vi "PID_Tank.vi"() -> ()   [LabVIEW 2014]
uses:
  <vilib>/Simulation/Scripting/Companion Diagram/SimConfigNode/SimParams.ctl
  <vilib>/Simulation/Scripting/Companion Diagram/SimConfigNode/_simSolvers.ctl
  <vilib>/Simulation/Implementation/Shared/SIMSCR Execution Mode.ctl
  <vilib>/Simulation/Param Hierarchy/Typedefs/SIMPH Param Control Actions.ctl
  <vilib>/Simulation/Implementation/Shared/SIM limit type.ctl
  <vilib>/Simulation/Implementation/Shared/NILVSim_ParamChanged.vi
  <vilib>/Simulation/Implementation/Shared/NILVSIM_BeginStep.vi
  <vilib>/Simulation/DataSources/Implementation/NILVSim Step.llb/SIM Step (scalar).vi
  <vilib>/Simulation/ContinuousLinear/Implementation/NILVSim Transport Delay.llb/SIM Transport Delay Distributor (scalar).vi
  <vilib>/Simulation/ContinuousLinear/Implementation/NILVSim Integrator new.llb/SIM Integrator distributor (scalar).vi
  <vilib>/Simulation/ContinuousLinear/Implementation/NILVSim Integrator new.llb/SIM Integrator collector (scalar).vi
  <vilib>/Simulation/ContinuousLinear/Implementation/NILVSim Derivative.llb/SIM derivative (scalar).vi
  <vilib>/Simulation/ContinuousLinear/Implementation/NILVSim Transport Delay.llb/SIM Transport Delay Collector (scalar).vi
  <vilib>/Simulation/SignalDisplay/Implementation/NILVSim Time Waveform.llb/SIM Time Waveform (vector).vi
  <vilib>/Simulation/Implementation/Shared/NILVSim_Manager.vi
  <vilib>/Utility/error.llb/Clear Errors.vi
  <vilib>/Simulation/Implementation/Shared/NILVSim_FinalizeModel.vi
  <vilib>/Simulation/Implementation/Shared/SIM Unbundle Sim Info.vi
  <vilib>/Simulation/Implementation/Shared/SIMSH Read Queue.vi
  <vilib>/Simulation/Implementation/Shared/NILVSim_Initialize.vi
  <vilib>/Simulation/Utility/Implementation/NILVSim Get Time and IsAcceptedStep.vi
  <vilib>/Simulation/Implementation/Shared/NILVSim_GetModelError.vi
  <vilib>/Simulation/Implementation/Shared/SIM Bundle Sim Info.vi
  <vilib>/Simulation/Scripting/Companion Diagram/SimConfigNode/SimDog.xnode
  <vilib>/Simulation/Implementation/XNodeFramework/SimXNode/SimX.xnode
  <vilib>/Simulation/ContinuousLinear/Implementation/NILVSim Integrator new.llb/SIM Integrator (scalar).vi
  <vilib>/Simulation/ContinuousLinear/Implementation/NILVSim Transport Delay.llb/SIM Transport Delay Indirect (scalar).vi
  <vilib>/Simulation/Implementation/Shared/NI_SIM_Implementation.lvlib
panel:
  in  "Flujo inicial en tuberia":dbl=2.0
  in  "H0":dbl=2.0
  in  "Href":dbl=2.0
  out "Valvula-2":dbl
  out "Perturbacion":dbl caption="ISE 2"
  in  "factor Ti2":dbl=1.0
  out "Tank  Control AMIGO":dbl(slide) scale=0.0..2.0
  in  "factor Td2":dbl=1.0
  in  "factor Kc2":dbl=1.0
  out "ISE 2":dbl
  out "ISE 1":dbl
  out "Valvulas":waveform(dbl)[](graph)
  in  "factor Kc1":dbl=1.0
  in  "factor Td1":dbl=1.0
  in  "Amplitud perturbacion":dbl=0.1
  out "Td2":dbl
  out "Ti2":dbl
  out "Kc2":dbl
  out "Td1":dbl
  out "Ti1":dbl
  out "Kc1":dbl
  in  "tp":dbl=30.5
  in  "Tt":dbl=7.4
  in  "Kp":dbl=68.3
  out "ISE":waveform(dbl)[](graph)
  out "Tank Control ZN O.L.":dbl(slide) scale=0.0..2.0
  in  "K1":dbl=1.21
  in  "A1":dbl=2.0
  in  "factor Ti1":dbl=1.0
  out "Alturas":waveform(dbl)[](graph)
  # "Dise–o de controladores de altura de un dep—sito"
  # "Altura de Referencia"
  # "PERTURBACIîN"
  # "CONTROLADORES PID"
  # "SISTEMA"
  # "IDENTIFICACIîN"
  # "Ziegler-Nichols O.L."
  # "AMIGO"
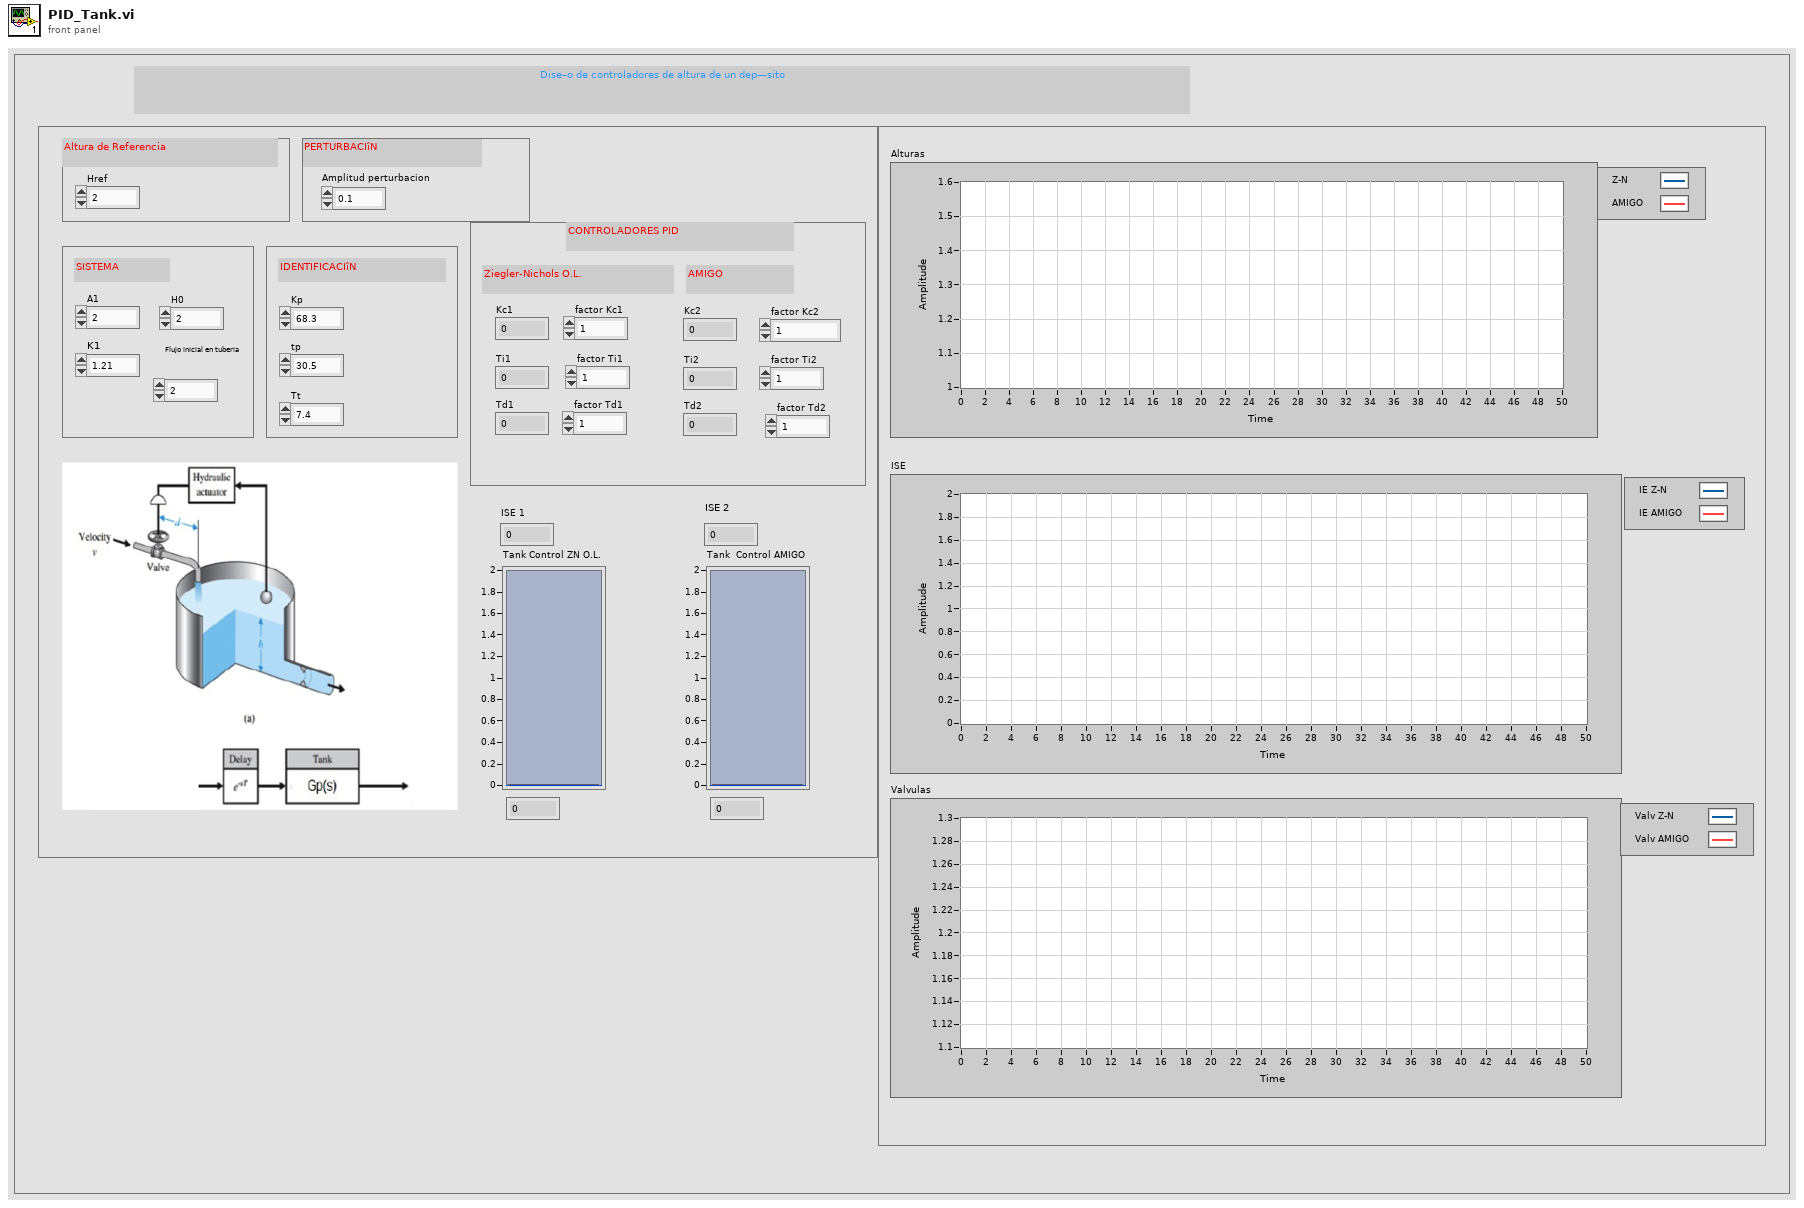
[diagram p1: front panel]
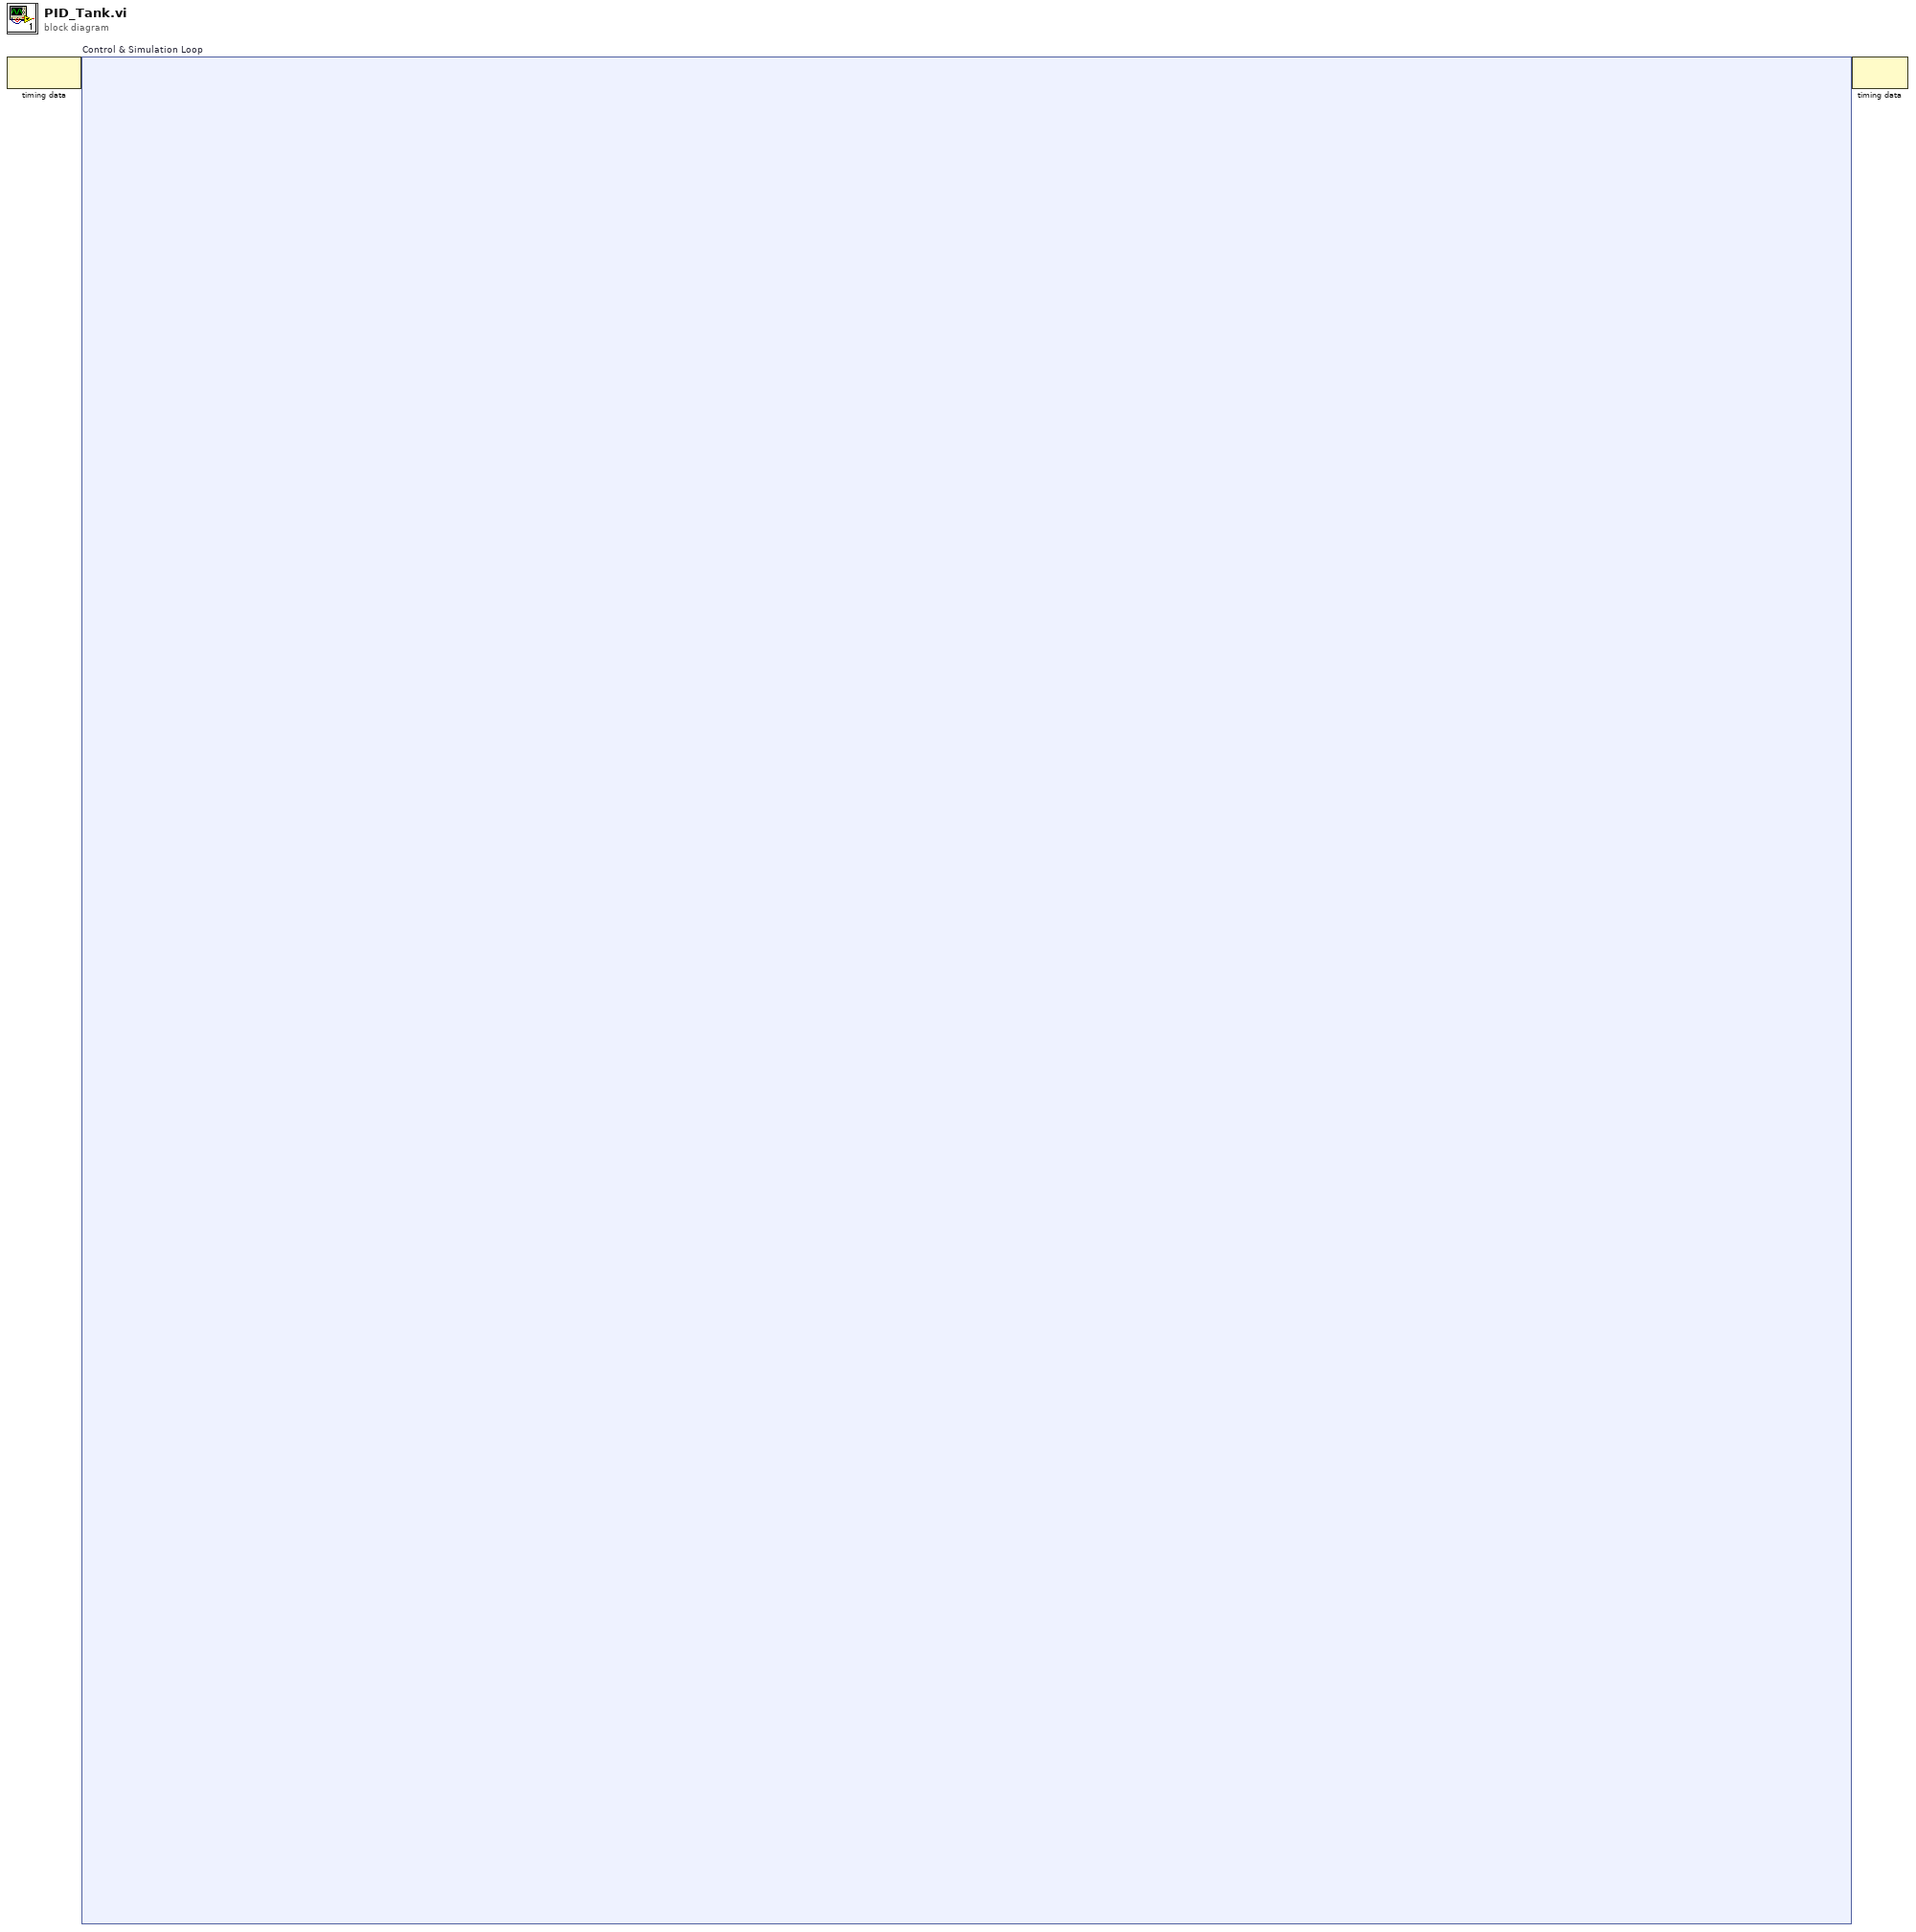
[diagram p0: block diagram]
diagram:
  n1 = node-c288() -> (w2:variant)  [unwired: 1 in]
  n2 = node-c254 "Control & Simulation Loop"(w2) -> (w1:variant)
  n3 = node-c288(w1) -> ()  [unwired: 1 out]
